vi "Set Task Setpoint.vi"(7 "Task Ident":string, 8 "error in":errorcluster, 9 "Data":variant, 10 "Setpoint Ident":string, 11 "Series Actor in":refnum<class "Series Actor.lvclass">) -> (0 "error out":errorcluster, 3 "Series Actor out":refnum<class "Series Actor.lvclass">)   [LabVIEW 2024, in "Series Actor.lvlib" / "Series Actor.lvclass"]
uses:
  Series Actor.lvclass
  Series Actor.lvclass/Series Actor.ctl
  Task/ITask Actor/ITask Actor Messages/Set Setpoint Msg/Set Setpoint Msg.lvclass/Set Setpoint Msg.ctl
  <vilib>/ActorFramework/Message Enqueuer/Message Enqueuer.lvclass/Message Enqueuer.ctl
  <vilib>/ActorFramework/Message Enqueuer/Enqueue.vi
  Task/ITask Actor/ITask Actor Messages/Set Setpoint Msg/Set Setpoint Msg.lvclass
  <vilib>/Utility/LVClass/Get LV Class Name.vi
  <resource>/AFDebug/Generate Trace for Message.vi
  <vilib>/ActorFramework/Message Priority Queue/Priority Enqueue.vi
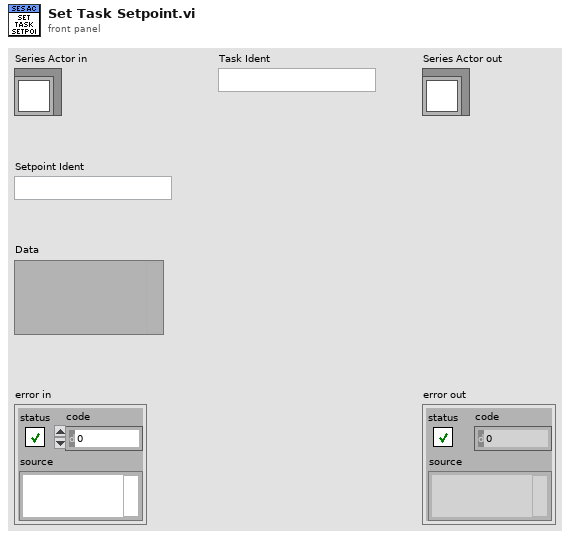
[diagram p1: front panel]
types:
  T1 = map{string, refnum<class "Message Enqueuer.lvclass">}
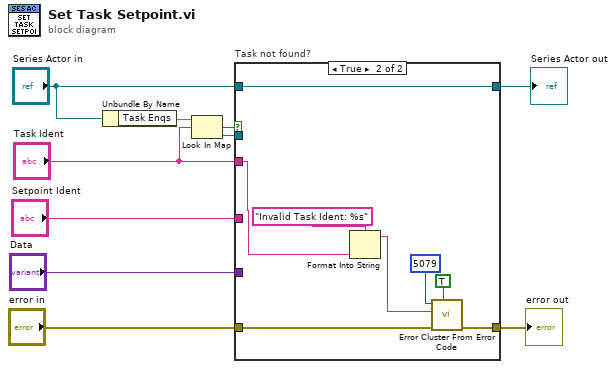
[diagram p0: block diagram]
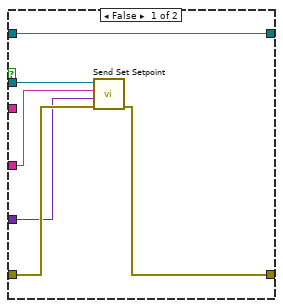
[diagram p2: hidden frame]
diagram:
  n1 = Unbundle By Name("Series Actor in") -> ("Task Enqs"=w10:T1)
  n2 = Look In Map(map=w10, key="Task Ident") -> (key not found?=w9:bool, value=w8:refnum<class "Message Enqueuer.lvclass">)  [unwired: 1 in]
  n3 = case "Task not found?" shown="True" w9 {
    tunnel: w8 -> [w16 _]
    tunnel: "Data" -> [w13 _]
    tunnel: [w12 w24] -> w4
    tunnel: "Setpoint Ident" -> [w11 _]
    tunnel: "error in" -> [w15 w19]
    tunnel: "Task Ident" -> [_ w18]
    tunnel: "Series Actor in" -> [w14 w17]
    tunnel: [w14 w17] -> w1
    frame False {
      n4 = call "Send Set Setpoint.vi"("error in (no error)"=w15, "Data"=w13, "Ident"=w11, "Message Enqueuer"=w16) -> ("error out"=w12:errorcluster)  [unwired: 6 in, 1 out]
    }
    frame True {
      n5 = Format Into String(format string="Invalid Task Ident: %s", w18) -> (resulting string=w20:string)  [unwired: 2 in, 1 out]
      n6 = call <vilib>:"Error Cluster From Error Code.vi"("show call chain? (False)"=TRUE, "error in (no error)"=w19, "error message (\"\")"=w20, "error code (0)"=5079) -> ("error out"=w24:errorcluster)  [unwired: 5 in]
    }
  }
  "error out" <- w4
  "Series Actor out" <- w1
